vi "Test Reset Triggers Broadcast.vi"(8 "error in (no error)":errorcluster, 11 "Test Case In":refnum<class "Debugger Test.lvclass">) -> (0 "error out":errorcluster, 3 "Test Case Out":refnum<class "Debugger Test.lvclass">)   [LabVIEW 2020, in "Debugger Test.lvclass"]
uses:
  Debugger Test.lvclass
  Debugger Test.lvclass/Debugger Test.ctl
  01074fa8-ee8a-411d-bc8b-fc92c4f90959.vi
  source/Process/Debug Process.lvclass
  source/Debugger/Debugger.lvclass
  source/Debug Data/Debug Data.lvclass
  source/Debug Data/Raw Debug Data.ctl
  C:/Users/anton/Documents/GitHub/triarc-debugger/source/Process/Debug Process.lvclass
  C:/Users/anton/Documents/GitHub/triarc-debugger/source/Debugger/Debugger.lvclass
  C:/Users/anton/Documents/GitHub/triarc-debugger/source/Debug Data Event/Debug Data Listener.lvclass
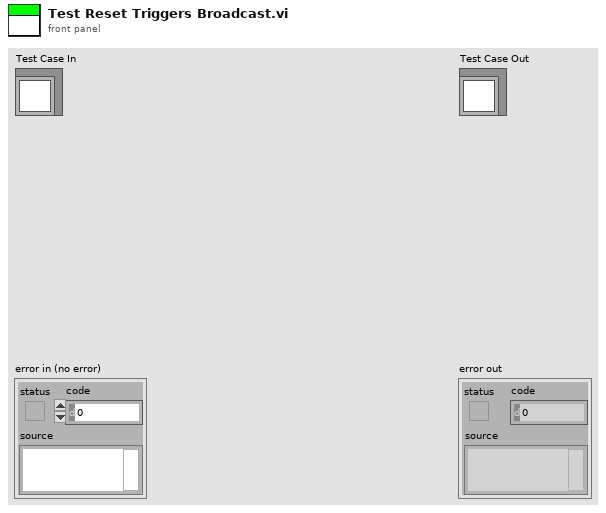
[diagram p1: front panel]
types:
  T1 = typedef "Debug Data.lvclass/Raw Debug Data.ctl" = cluster{"Action":string, "Call Chain":string, "Process":string, "Message":string, "Message Data":variant, "Time":dbl}
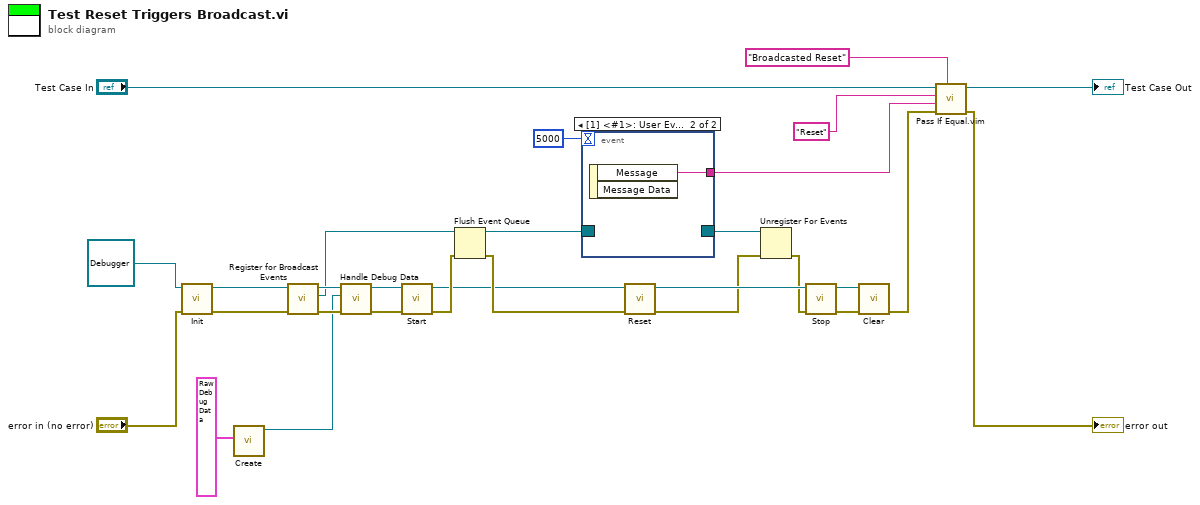
[diagram p0: block diagram]
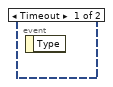
[diagram p2: hidden frame]
diagram:
  n1 = call-dynamic "Init.vi"("error in (no error)"="error in (no error)", "Process In"=refnum<class "Debugger.lvclass"> refnum ("Debug Data Event In 2")) -> ("error out"=w7:errorcluster, "Process Out"=w8:refnum<class "Debugger.lvclass">)  [unwired: 8 in]
  n2 = call "Create.vi"("Debug Data Cluster"=T1 {"Action"="", "Call Chain"="", "Process"="Test", "Message"="", "Message Data"=variant, "Time"=0.0}) -> ("Debug Data out"=w15:refnum<class "Debug Data.lvclass">)  [unwired: 9 in, 1 out]
  n3 = call "Register for Broadcast Events.vi"("error in (no error)"=w7, "Process In"=w8) -> ("error out"=w26:errorcluster, "Event Registration Refnum Out"=w13:refnum<event-registration>, "Process Out"=w22:refnum<class "Debugger.lvclass">)  [unwired: 7 in]
  n4 = call-dynamic "Handle Debug Data.vi"("error in (no error)"=w26, "Debug Data.lvclass"=w15, "Debug Data Event In"=w22) -> ("error out"=w6:errorcluster, "Debug Data Event Out"=w4:refnum<class "Debugger.lvclass">)  [unwired: 7 in]
  n5 = call "Start.vi"("error in (no error)"=w6, "Process In"=w4) -> ("error out"=w5:errorcluster, "Process Out"=w3:refnum<class "Debugger.lvclass">)  [unwired: 7 in, 1 out]
  n6 = Flush Event Queue(0:w13, 3:w5) -> (8:w12:refnum<event-registration>, 11:w14:errorcluster)  [unwired: 4 in, 1 out]
  n7 = event shown="[1] <#1>: User Event" {
    selector: w12 -> [_ _]
    dyn-events: [_ _] -> w17
    timeout: 5000 -> [_ _]
    tunnel: [_ w30] -> w2
    event Timeout {
      n8 = event-data() -> ()  [unwired: 1 in, 1 out]
    }
    event User Event {
      n9 = event-data() -> ("Message"=w30:string)  [unwired: 1 in, 1 out]
    }
  }
  n10 = call "Reset.vi"("error in (no error)"=w14, "Debugger in"=w3) -> ("error out"=w9:errorcluster, "Debugger out"=w25:refnum<class "Debugger.lvclass">)  [unwired: 8 in]
  n11 = Unregister For Events(event registration refnum=w17, error in=w9) -> (error out=w10:errorcluster)
  n12 = call "Stop.vi"("error in (no error)"=w10, "Process In"=w25) -> ("error out"=w23:errorcluster, "Process Out"=w24:refnum<class "Debugger.lvclass">)  [unwired: 7 in, 1 out]
  n13 = call-dynamic "Clear.vi"("error in (no error)"=w23, "Process In"=w24) -> ("error out"=w11:errorcluster)  [unwired: 9 in]
  n14 = call "Pass If Equal.vim"("Description"="Broadcasted Reset", "error in (no error)"=w11, "Actual"=w2, "Expected"="Reset", "LUnit Test Case In"="Test Case In") -> ("error out"=→"error out":errorcluster, "LUnit Test Case Out"=→"Test Case Out":refnum<class "Debugger Test.lvclass">)  [unwired: 5 in]
